vi "Pot Home Values.vi"() -> ()   [LabVIEW 2012]
panel:
  in  "Pot Home Values":dbl[](array[numeric])
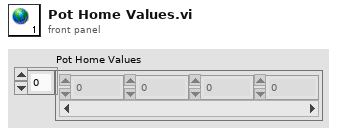
[diagram p1: front panel]
diagram:
